vi "classification to display permissions.vi"(11 "channel classification":T1) -> (3 "permissions":T2)   [LabVIEW 2013, in "TEC editor node.lvclass"]
uses:
  TEC editor node.lvclass
  permissions.ctl
  <vilib>/NI/Tag Bus Module Framework/channel/channel classification.ctl
  <vilib>/NI/Tag Bus Module Framework/channel/TBM channel.lvclass
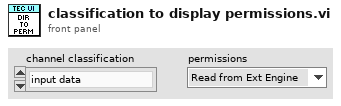
[diagram p1: front panel]
types:
  T1 = typedef "TBM channel.lvclass/channel classification.ctl" = enum16{"input data", "output data", "processing parameter", "processing result"}
  T2 = typedef "TEC editor node.lvclass/permissions.ctl" = enum16{"Read from Ext Engine", "Write to Ext Engine"}
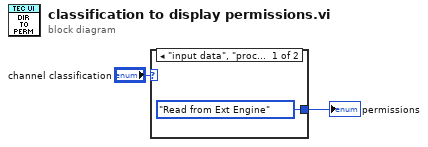
[diagram p0: block diagram]
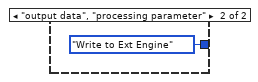
[diagram p2: hidden frame]
diagram:
  n1 = case shown="\"input data\", \"processing result\"" "channel classification" {
    tunnel: [permissions."Read from Ext Engine" ("permissions") permissions."Write to Ext Engine" ("permissions")] -> w2
    frame "input data", "processing result" {
    }
    frame "output data", "processing parameter" {
    }
  }
  "permissions" <- w2
